vi "Auto Calibrate.vi"(8 "error in (no error)":errorcluster, 11 "Optical Spectrum Analyzer in":refnum<class "Optical Spectrum Analyzer.lvclass">) -> (0 "error out":errorcluster, 3 "Optical Spectrum Analyzer out":refnum<class "Optical Spectrum Analyzer.lvclass">)   [LabVIEW 2018, in "Optical Spectrum Analyzer.lvlib" / "Optical Spectrum Analyzer.lvclass"]
uses:
  Optical Spectrum Analyzer.lvclass
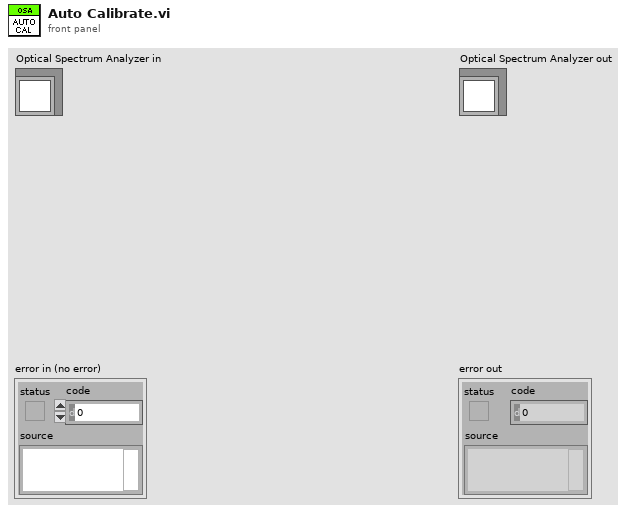
[diagram p1: front panel]
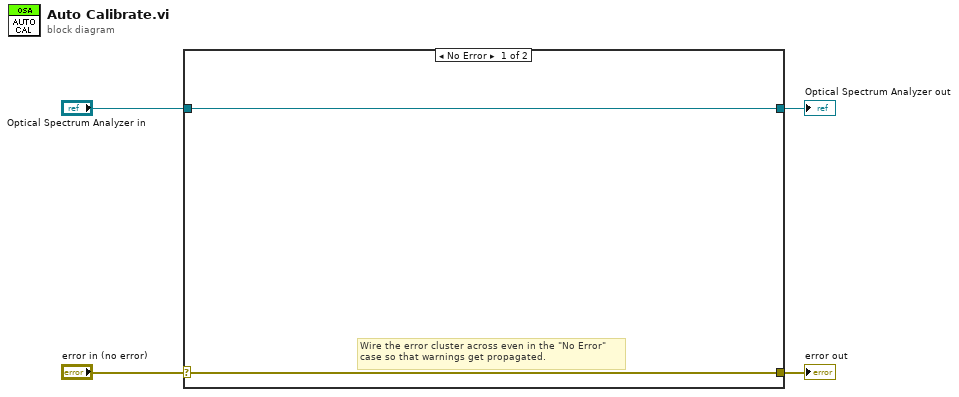
[diagram p0: block diagram]
diagram:
  n1 = case shown="No Error" "error in (no error)" {
    selector: "error in (no error)" -> [w5 w8]
    tunnel: [w5 w8] -> w3
    tunnel: [w6 w7] -> w1
    tunnel: "Optical Spectrum Analyzer in" -> [w6 w7]
    frame No Error {
      # "Wire the error cluster across even in the \"No Error\"\ncase so that warnings get propagated."
    }
    frame Error {
    }
  }
  "error out" <- w3
  "Optical Spectrum Analyzer out" <- w1
